vi "Test ReInit.vi"(7 "Sequence Context In":refnum<k7>, 8 "error in":errorcluster, 9 "Test Mode":u16, 10 "LV PPS Config":T1={"VISA Resource"="", "Voltage Level (0.0 V)"=12.0, "CURRent Limit (0.0 A)"=6.0, "OVP LEVEL (0V)"=15.0, "Enable OVP (T: Enable)"=FALSE, "OCP LEVEL (0A)"=8.0, "Enable OCP (T: Enable)"=TRUE, "Value Out"="", "Value In"="", "Actual Voltage Level (V)"=-0.11, "Actual Current Limit (A)"=0.0, "Select Instrument"="", "Enable Output"=TRUE, "PPS Operation"=enum."Configure", "Type"=0} {"Type" items=["Voltage", "Current"]; "Actual Current Limit (A)" format="%.2f"; "Actual Voltage Level (V)" format="%.2f"; "OCP LEVEL (0A)" format="%.2f"; "OVP LEVEL (0V)" format="%.2f"; "Voltage Level (0.0 V)" format="%.2f"}, 11 "HV PPS Config":T1={"VISA Resource"="", "Voltage Level (0.0 V)"=48.0, "CURRent Limit (0.0 A)"=150.0, "OVP LEVEL (0V)"=55.0, "Enable OVP (T: Enable)"=FALSE, "OCP LEVEL (0A)"=160.0, "Enable OCP (T: Enable)"=TRUE, "Value Out"="", "Value In"="", "Actual Voltage Level (V)"=-0.11, "Actual Current Limit (A)"=0.0, "Select Instrument"="", "Enable Output"=TRUE, "PPS Operation"=enum."Configure", "Type"=0} {"Type" items=["Voltage", "Current"]; "Actual Current Limit (A)" format="%.2f"; "Actual Voltage Level (V)" format="%.2f"; "OCP LEVEL (0A)" format="%.2f"; "OVP LEVEL (0V)" format="%.2f"; "Voltage Level (0.0 V)" format="%.2f"}) -> (0 "error out":errorcluster, 2 "Response Code":u8[](array[numeric]), 3 "Positive Responce":bool)   [LabVIEW 2023, in "HardwareAbstractionLayer_LVOOP.lvlib" / "Wait Monitor.lvclass"]
uses:
  Wait Monitor.lvclass
  PowerSupply/Teststand/Control/PPS StepType Control.ctl
  CAN/CAN Application Protocols/STP Protocol_class/Ctrls/STP CMD.ctl
  Teststand Steptypes/CAN/STP/Steptypes/Control/STP Data.ctl
  Teststand Steptypes/DAQ/Relay Output/Control/Relay Output.ctl
  069355f8-7d87-48c7-8f90-e89c4997140f.vi
  3c8db822-b366-47eb-99a2-87ce3c109eb2.vi
  f5ace3f9-55e8-4b56-8f2c-1356bb897dc4.vi
  57b82cc3-dd7c-4d3a-8ba9-81b38abffcad.vi
  725d82db-e125-4af1-8c31-2eddca650097.vi
  e56fdc52-0104-40be-a5d4-315e7d7fad48.vi
  ae1cdcb4-d38d-44ac-ba66-047396e49866.vi
  Teststand/Teststand.lvclass
  PowerSupply/PowerSupply.lvclass
  CAN/CAN Application Protocols/STP Protocol_class/STP Protocol.lvclass
  Teststand Steptypes/LTT_TeststandSteptypes.lvlib
  b7294423-ed5d-4e5b-8d0b-fca4433a2c56.vi
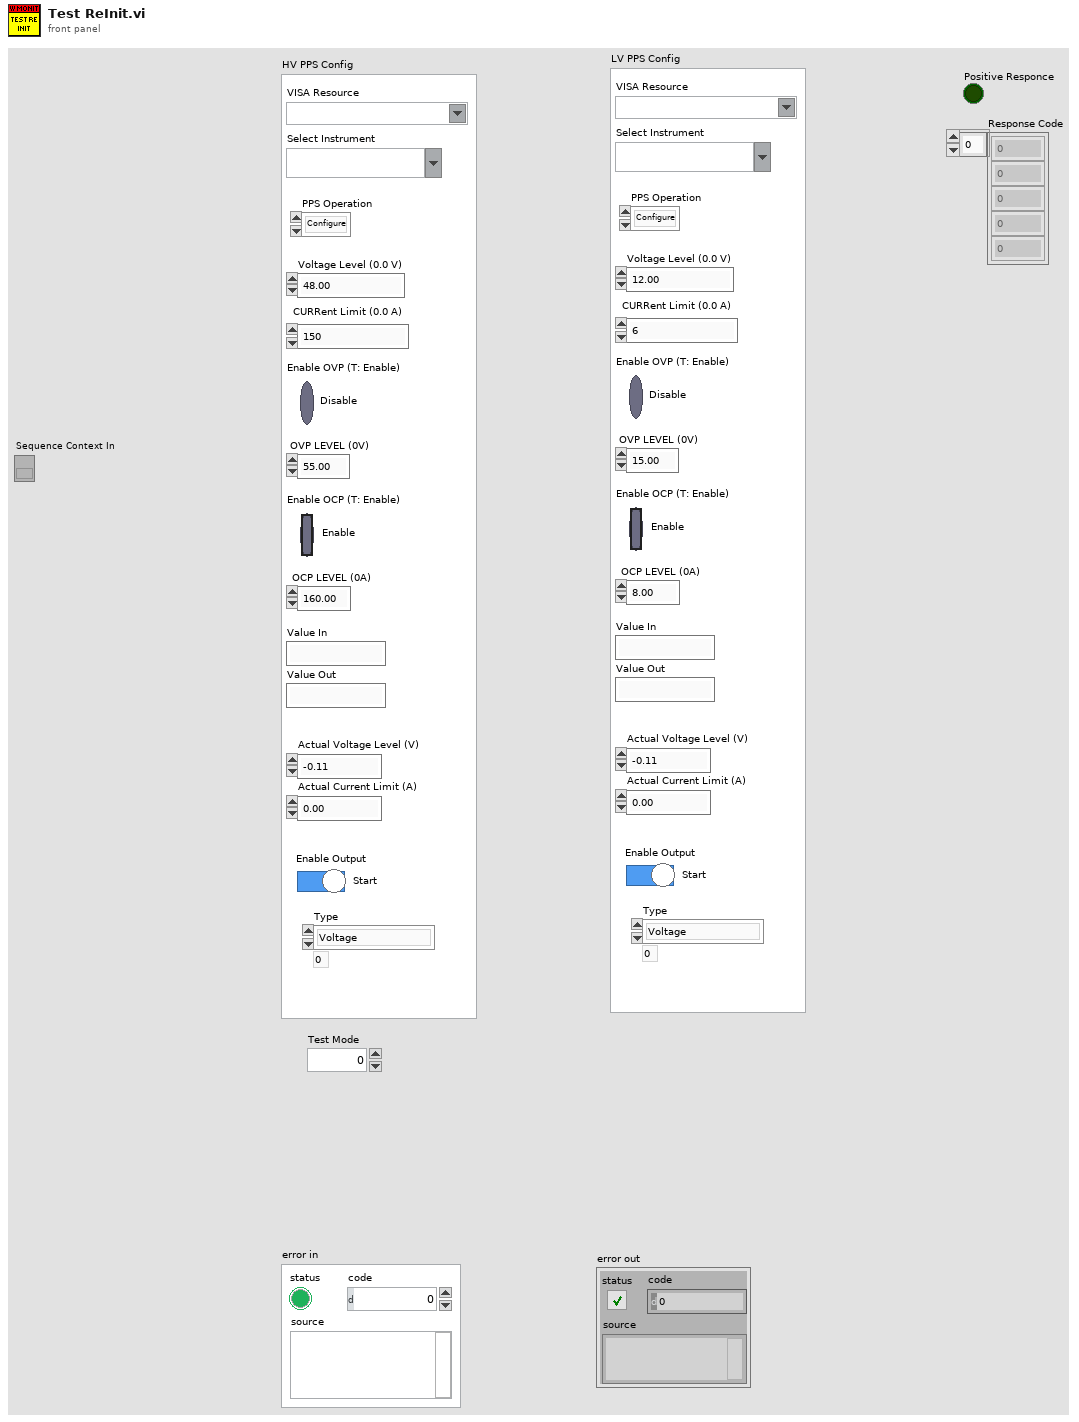
[diagram p1: front panel]
types:
  T1 = typedef "HardwareAbstractionLayer_LVOOP.lvlib/PowerSupply.lvclass/PPS StepType Control.ctl" = cluster{"VISA Resource":refnum<visa-resource-name>, "Voltage Level (0.0 V)":dbl, "CURRent Limit (0.0 A)":dbl, "OVP LEVEL (0V)":dbl, "Enable OVP (T: Enable)":bool, "OCP LEVEL (0A)":dbl, "Enable OCP (T: Enable)":bool, "Value Out":string, "Value In":string, "Actual Voltage Level (V)":dbl, "Actual Current Limit (A)":dbl, "Select Instrument":string, "Enable Output":bool, "PPS Operation":enum32{"Init", "Self Test", "Configure", "Measure", "Close"}, "Type":u16}
  T2 = enum32{"Init", "Self Test", "Configure", "Measure", "Close"}
  T3 = typedef "LTT_TeststandSteptypes.lvlib/STP Data.ctl" = cluster{"ECU CAN Port":string, "CMD":T4, "CAN Write Data":u8[], "Response Decoder":enum16{"String", "Number", "Boolean"}, "String":cluster{"Start Index":i32, "Length":i32}, "Number":cluster{"MSB Index":i32, "LSB Index":i32}, "Boolean":cluster{"Index":i32, "Bool":cluster{"7":bool, "6":bool, "5":bool, "4":bool, "3":bool, "2":bool, "1":bool, "0":bool, "7 Enabled":bool, "6 Enabled":bool, "5 Enabled":bool, "4 Enabled":bool, "3 Enabled":bool, "2 Enabled":bool, "1 Enabled":bool, "0 Enabled":bool}}}
  T4 = typedef "HardwareAbstractionLayer_LVOOP.lvlib/CAN Application Protocols Lib.lvlib/STP Protocol.lvclass/STP CMD.ctl" = u8
  T5 = typedef "LTT_TeststandSteptypes.lvlib/Relay Output.ctl" = cluster{"Signal Name List":cluster{"Signal Name":string, "Enable Output":bool}[]}
  T6 = typedef "HardwareAbstractionLayer_LVOOP.lvlib/Teststand.lvclass/Teststand Status Control.ctl" = cluster{"Terminating or Aborting":bool, "Stop":bool, "Socket Count":i16, "Selected Sockets":i16[]}
  T7 = typedef "LTT_TeststandSteptypes.lvlib/STP Out Data.ctl" = cluster{"String Data":string, "Numeric Data":dbl, "Boolean Data":bool, "RequestTimeout?":bool, "ResponseData":u8[], "PositiveResponse?":bool}
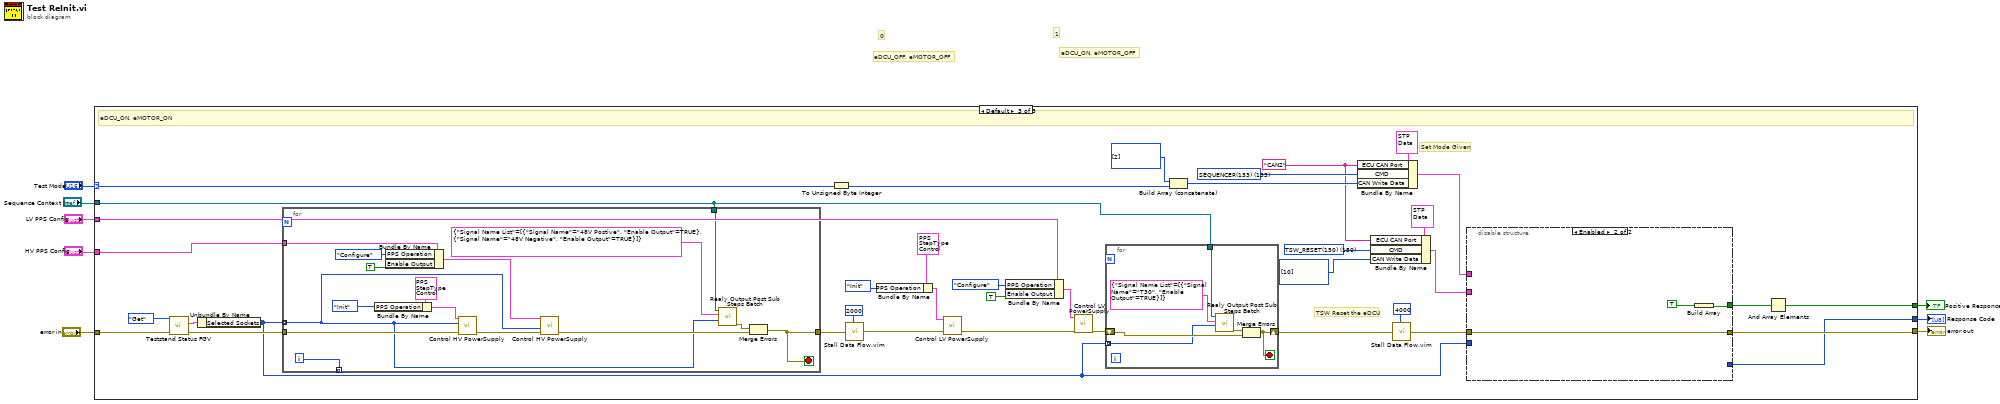
[diagram p0: block diagram]
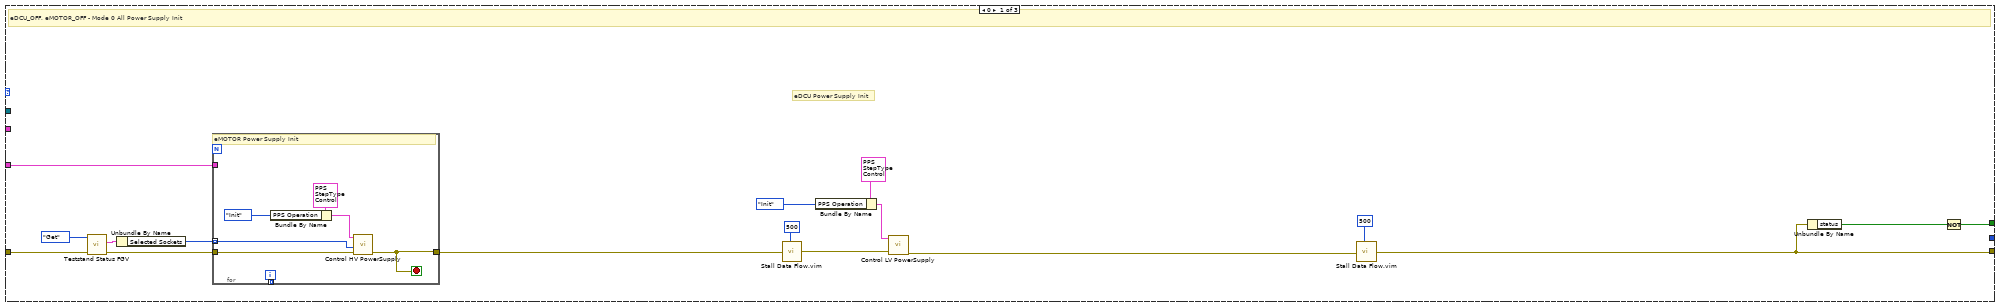
[diagram p2: hidden frame]
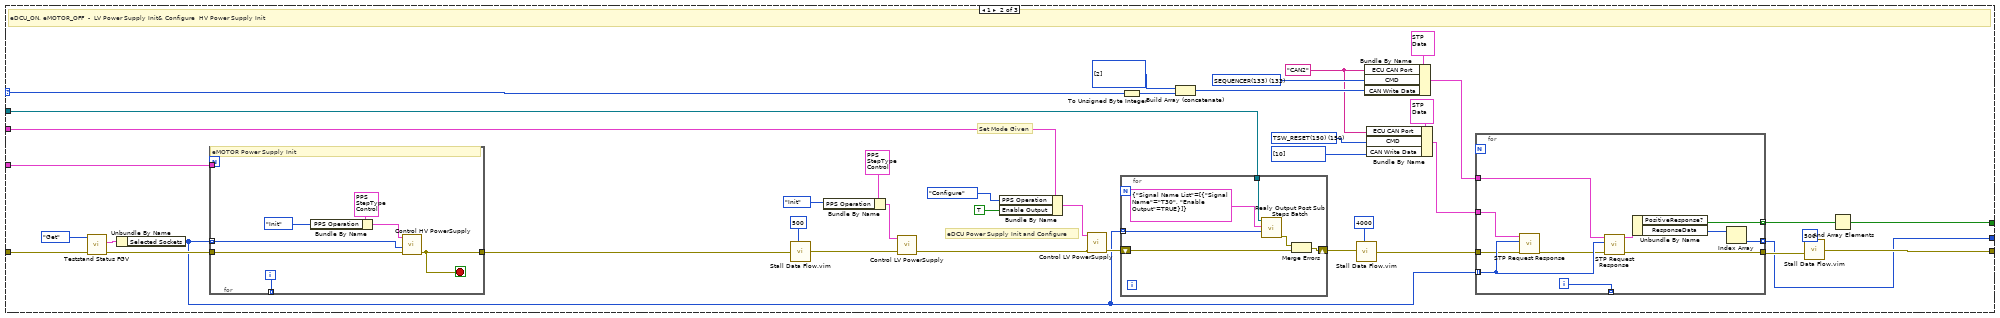
[diagram p3: hidden frame]
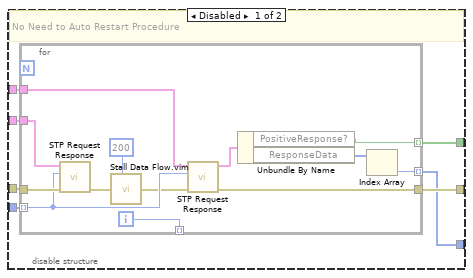
[diagram p4: hidden frame]
diagram:
  # "0"
  # "1"
  # "eDCU_ON, eMOTOR_OFF"
  # "eDCU_OFF, eMOTOR_OFF"
  n1 = case shown="Default" "Test Mode" {
    selector: "Test Mode" -> [_ w54 w116]
    tunnel: "error in" -> [w22 w69 w131]
    tunnel: [w11 w50 w122] -> w7
    tunnel: "HV PPS Config" -> [w21 w68 w130]
    tunnel: "LV PPS Config" -> [_ w63 w125]
    tunnel: [w10 w48 w112] -> w3
    tunnel: [_ w47 w111] -> w2
    tunnel: "Sequence Context In" -> [_ w38 w103]
    frame 0 {
      # "eDCU Power Supply Init"
      # "eDCU_OFF, eMOTOR_OFF - Mode 0 All Power Supply Init"
      n2 = call "Teststand Status FGV.vi"("error in"=w22, "Option"=enum16{"Set", "Get"}."Get") -> ("error out"=w23:errorcluster, "Teststand Status Out"=w24:T6)  [unwired: 8 in]
      n3 = Unbundle By Name(w24) -> ("Selected Sockets"=w15:i16[])
      n4 = for {
        tunnel: w23 -> [w31]
        tunnel: [w30] -> w20
        tunnel: w15 -> [w32] mode=indexing
        tunnel: w21 -> [_]
        tunnel: [w26] -> _ mode=indexing
        i -> [w26]
        stop <- w30 stop-if-true
        # "eMOTOR Power Supply Init"
        n5 = Bundle By Name(cluster=T1 {"VISA Resource"="", "Voltage Level (0.0 V)"=0.0, "CURRent Limit (0.0 A)"=0.0, "OVP LEVEL (0V)"=0.0, "Enable OVP (T: Enable)"=TRUE, "OCP LEVEL (0A)"=0.0, "Enable OCP (T: Enable)"=TRUE, "Value Out"="", "Value In"="", "Actual Voltage Level (V)"=0.0, "Actual Current Limit (A)"=0.0, "Select Instrument"="", "Enable Output"=FALSE, "PPS Operation"=enum."Init", "Type"=0} ("PPS Config In"), "PPS Operation"=T2."Init") -> (w27:T1)
        n6 = call "Control HV PowerSupply.vi"("error in"=w31, "Socket Index"=w32, "PPS Config In"=w27) -> ("error out"=w30:errorcluster)  [unwired: 6 in, 2 out]
      }
      n7 = call "Stall Data Flow.vim"("value in"=w20, "milliseconds to wait"=u32 500) -> ("value out"=w13:errorcluster)  [unwired: 1 out]
      n8 = Bundle By Name(cluster=T1 {"VISA Resource"="", "Voltage Level (0.0 V)"=12.0, "CURRent Limit (0.0 A)"=6.0, "OVP LEVEL (0V)"=15.0, "Enable OVP (T: Enable)"=FALSE, "OCP LEVEL (0A)"=8.0, "Enable OCP (T: Enable)"=TRUE, "Value Out"="", "Value In"="", "Actual Voltage Level (V)"=-0.11, "Actual Current Limit (A)"=0.0, "Select Instrument"="", "Enable Output"=TRUE, "PPS Operation"=enum."Init", "Type"=0} ("PPS Config In"), "PPS Operation"=T2."Init") -> (w14:T1)
      n9 = call "Control LV PowerSupply.vi"("error in"=w13, "PPS Config In"=w14) -> ("error out"=w12:errorcluster)  [unwired: 7 in, 2 out]
      n10 = call "Stall Data Flow.vim"("value in"=w12, "milliseconds to wait"=u32 500) -> ("value out"=w11:errorcluster)  [unwired: 1 out]
      n11 = Unbundle By Name(w11) -> ("status"=w9:bool)
      n12 = Not(x=w9) -> (.not. x?=w10:bool)
    }
    frame 1 {
      w36 = T4 150 items=["TSW_VERSION(130)"=130, "WAIT_EVENT(132)"=132, "SEQUENCER(133)"=133, "TSW_RESET(150)"=150, "CONFIG_ECU(151)"=151, "TEST_CORE (152)"=152, "TEST_WATCHDOG (153)"=153, "TEST_MONITORING (154)"=154, "READ_MEMORY (162)"=162, "WRITE_ERASE_MEMORY (164)"=164, "COMM_EXTERNAL (190)"=190, "COMM_INTERNAL (195)"=195, "GET_ANALOG_INPUT (210)"=210, "GET_DIGITAL_INPUT (211)"=211, "GET_FREQUENCY_INPUT (212)"=212, "TEST_INPUT_STRUCTURE (214)"=214, "GENERATE_OUTPUT_SIGNAL (220)"=220, "GENERATE_SYNCHRONIZED_OUTPUT_SIGNALS (221)"=221, "eDCU_Specific (250)"=250] ("CMD")
      w56 = T4 133 items=["TSW_VERSION(130)"=130, "WAIT_EVENT(132)"=132, "SEQUENCER(133)"=133, "TSW_RESET(150)"=150, "CONFIG_ECU(151)"=151, "TEST_CORE (152)"=152, "TEST_WATCHDOG (153)"=153, "TEST_MONITORING (154)"=154, "READ_MEMORY (162)"=162, "WRITE_ERASE_MEMORY (164)"=164, "COMM_EXTERNAL (190)"=190, "COMM_INTERNAL (195)"=195, "GET_ANALOG_INPUT (210)"=210, "GET_DIGITAL_INPUT (211)"=211, "GET_FREQUENCY_INPUT (212)"=212, "TEST_INPUT_STRUCTURE (214)"=214, "GENERATE_OUTPUT_SIGNAL (220)"=220, "GENERATE_SYNCHRONIZED_OUTPUT_SIGNALS (221)"=221, "eDCU_Specific (250)"=250] ("CMD")
      w35 = "CAN2" ("ECU CAN Port")
      # "eDCU Power Supply Init and Configure"
      # "Set Mode Given"
      # "eDCU_ON, eMOTOR_OFF  -  LV Power Supply Init& Configure  HV Power Supply Init"
      n13 = call "Teststand Status FGV.vi"("error in"=w69, "Option"=enum16{"Set", "Get"}."Get") -> ("error out"=w70:errorcluster, "Teststand Status Out"=w71:T6)  [unwired: 8 in]
      n14 = Unbundle By Name(w71) -> ("Selected Sockets"=w39:i16[])
      n15 = for {
        tunnel: w70 -> [w95]
        tunnel: [w94] -> w67
        tunnel: w39 -> [w96] mode=indexing
        tunnel: w68 -> [_]
        tunnel: [w90] -> _ mode=indexing
        i -> [w90]
        stop <- w94 stop-if-true
        # "eMOTOR Power Supply Init"
        n16 = Bundle By Name(cluster=T1 {"VISA Resource"="", "Voltage Level (0.0 V)"=0.0, "CURRent Limit (0.0 A)"=0.0, "OVP LEVEL (0V)"=0.0, "Enable OVP (T: Enable)"=TRUE, "OCP LEVEL (0A)"=0.0, "Enable OCP (T: Enable)"=TRUE, "Value Out"="", "Value In"="", "Actual Voltage Level (V)"=0.0, "Actual Current Limit (A)"=0.0, "Select Instrument"="", "Enable Output"=FALSE, "PPS Operation"=enum."Init", "Type"=0} ("PPS Config In"), "PPS Operation"=T2."Init") -> (w91:T1)
        n17 = call "Control HV PowerSupply.vi"("error in"=w95, "Socket Index"=w96, "PPS Config In"=w91) -> ("error out"=w94:errorcluster)  [unwired: 6 in, 2 out]
      }
      n18 = call "Stall Data Flow.vim"("value in"=w67, "milliseconds to wait"=u32 500) -> ("value out"=w45:errorcluster)  [unwired: 1 out]
      n19 = Bundle By Name(cluster=T1 {"VISA Resource"="", "Voltage Level (0.0 V)"=12.0, "CURRent Limit (0.0 A)"=6.0, "OVP LEVEL (0V)"=15.0, "Enable OVP (T: Enable)"=FALSE, "OCP LEVEL (0A)"=8.0, "Enable OCP (T: Enable)"=TRUE, "Value Out"="", "Value In"="", "Actual Voltage Level (V)"=-0.11, "Actual Current Limit (A)"=0.0, "Select Instrument"="", "Enable Output"=TRUE, "PPS Operation"=enum."Init", "Type"=0} ("PPS Config In"), "PPS Operation"=T2."Init") -> (w46:T1)
      n20 = call "Control LV PowerSupply.vi"("error in"=w45, "PPS Config In"=w46) -> ("error out"=w43:errorcluster)  [unwired: 7 in, 2 out]
      n21 = Bundle By Name(cluster=w63, "PPS Operation"=T2."Configure", "Enable Output"=TRUE) -> (w44:T1)
      n22 = call "Control LV PowerSupply.vi"("error in"=w43, "PPS Config In"=w44) -> ("error out"=w41:errorcluster)  [unwired: 7 in, 2 out]
      n23 = for {
        tunnel: w38 -> [w77]
        shift-right: [w75] -> w40
        shift-left: w41 -> [w76]
        tunnel: w39 -> [w73] mode=indexing
        n24 = call "Realy Output Post Sub Steps Batch.vi"("Socket No"=w73, "RelayOutputWrite"=T5 {"Signal Name List"=[{"Signal Name"="T30", "Enable Output"=TRUE}]}, "Sequence Context In"=w77) -> ("error out"=w74:errorcluster)  [unwired: 6 in, 2 out]
        n25 = Merge Errors(w74, w76) -> (w75:errorcluster)
      }
      n26 = To Unsigned Byte Integer(number=w54) -> (unsigned 8bit integer=w53:u8)
      n27 = Build Array (concatenate)(u8[] [2] ("CAN Write Data"), w53) -> (w52:u8[])
      n28 = call "Stall Data Flow.vim"("value in"=w40, "milliseconds to wait"=u32 4000) -> ("value out"=w59:errorcluster)  [unwired: 1 out]
      n29 = Bundle By Name(cluster=T3 {"ECU CAN Port"="CAN2", "CMD"=130, "CAN Write Data"=[], "Response Decoder"=enum."String", "String"={"Start Index"=0, "Length"=-1}, "Number"={"MSB Index"=0, "LSB Index"=1}, "Boolean"={"Index"=0, "Bool"={"7"=FALSE, "6"=FALSE, "5"=FALSE, "4"=FALSE, "3"=FALSE, "2"=FALSE, "1"=FALSE, "0"=FALSE, "7 Enabled"=FALSE, "6 Enabled"=FALSE, "5 Enabled"=FALSE, "4 Enabled"=FALSE, "3 Enabled"=FALSE, "2 Enabled"=FALSE, "1 Enabled"=FALSE, "0 Enabled"=FALSE}}} ("STP Data in"), "ECU CAN Port"=w35, "CMD"=w56, "CAN Write Data"=w52) -> (w57:T3)
      n30 = Bundle By Name(cluster=T3 {"ECU CAN Port"="CAN2", "CMD"=130, "CAN Write Data"=[], "Response Decoder"=enum."String", "String"={"Start Index"=0, "Length"=-1}, "Number"={"MSB Index"=0, "LSB Index"=1}, "Boolean"={"Index"=0, "Bool"={"7"=FALSE, "6"=FALSE, "5"=FALSE, "4"=FALSE, "3"=FALSE, "2"=FALSE, "1"=FALSE, "0"=FALSE, "7 Enabled"=FALSE, "6 Enabled"=FALSE, "5 Enabled"=FALSE, "4 Enabled"=FALSE, "3 Enabled"=FALSE, "2 Enabled"=FALSE, "1 Enabled"=FALSE, "0 Enabled"=FALSE}}} ("STP Data in"), "ECU CAN Port"=w35, "CMD"=w36, "CAN Write Data"=u8[] [10]) -> (w33:T3)
      n31 = for {
        tunnel: w57 -> [w88]
        tunnel: [w87] -> _ mode=indexing
        tunnel: w39 -> [w82] mode=indexing
        tunnel: w59 -> [w80]
        tunnel: [w89] -> w60
        tunnel: [w85] -> w51 mode=indexing
        tunnel: [w83] -> w47 mode=indexing
        tunnel: w33 -> [w81]
        i -> [w87]
        n32 = call "STP Request Response.vi"("error in"=w80, "Socket No"=w82, "STP Data in"=w81) -> ("error out"=w79:errorcluster)  [unwired: 5 in, 3 out]
        n33 = call "STP Request Response.vi"("error in"=w79, "Socket No"=w82, "STP Data in"=w88) -> ("error out"=w89:errorcluster, "STP Data Out"=w86:T7)  [unwired: 5 in, 2 out]
        n34 = Unbundle By Name(w86) -> ("PositiveResponse?"=w85:bool, "ResponseData"=w84:u8[])
        n35 = Index Array(array=w84) -> (element=w83:u8)  [unwired: 1 in]
      }
      n36 = call "Stall Data Flow.vim"("value in"=w60, "milliseconds to wait"=u32 500) -> ("value out"=w50:errorcluster)  [unwired: 1 out]
      n37 = And Array Elements(Boolean array=w51) -> (logical AND=w48:bool)
    }
    frame Default {
      w100 = T4 150 items=["TSW_VERSION(130)"=130, "WAIT_EVENT(132)"=132, "SEQUENCER(133)"=133, "TSW_RESET(150)"=150, "CONFIG_ECU(151)"=151, "TEST_CORE (152)"=152, "TEST_WATCHDOG (153)"=153, "TEST_MONITORING (154)"=154, "READ_MEMORY (162)"=162, "WRITE_ERASE_MEMORY (164)"=164, "COMM_EXTERNAL (190)"=190, "COMM_INTERNAL (195)"=195, "GET_ANALOG_INPUT (210)"=210, "GET_DIGITAL_INPUT (211)"=211, "GET_FREQUENCY_INPUT (212)"=212, "TEST_INPUT_STRUCTURE (214)"=214, "GENERATE_OUTPUT_SIGNAL (220)"=220, "GENERATE_SYNCHRONIZED_OUTPUT_SIGNALS (221)"=221, "eDCU_Specific (250)"=250] ("CMD")
      w118 = T4 133 items=["TSW_VERSION(130)"=130, "WAIT_EVENT(132)"=132, "SEQUENCER(133)"=133, "TSW_RESET(150)"=150, "CONFIG_ECU(151)"=151, "TEST_CORE (152)"=152, "TEST_WATCHDOG (153)"=153, "TEST_MONITORING (154)"=154, "READ_MEMORY (162)"=162, "WRITE_ERASE_MEMORY (164)"=164, "COMM_EXTERNAL (190)"=190, "COMM_INTERNAL (195)"=195, "GET_ANALOG_INPUT (210)"=210, "GET_DIGITAL_INPUT (211)"=211, "GET_FREQUENCY_INPUT (212)"=212, "TEST_INPUT_STRUCTURE (214)"=214, "GENERATE_OUTPUT_SIGNAL (220)"=220, "GENERATE_SYNCHRONIZED_OUTPUT_SIGNALS (221)"=221, "eDCU_Specific (250)"=250] ("CMD")
      w97 = "CAN2" ("ECU CAN Port")
      # "TSW Reset the eDCU"
      # "Set Mode Given"
      # "eDCU_ON, eMOTOR_ON"
      n38 = call "Teststand Status FGV.vi"("error in"=w131, "Option"=enum16{"Set", "Get"}."Get") -> ("error out"=w132:errorcluster, "Teststand Status Out"=w133:T6)  [unwired: 8 in]
      n39 = Unbundle By Name(w133) -> ("Selected Sockets"=w102:i16[])
      n40 = for {
        tunnel: w132 -> [w175]
        tunnel: [w166] -> w129
        tunnel: w102 -> [w164] mode=indexing
        tunnel: w130 -> [w178]
        tunnel: [w170] -> _ mode=indexing
        tunnel: w103 -> [w167]
        i -> [w170]
        stop <- w166 stop-if-true
        n41 = Bundle By Name(cluster=T1 {"VISA Resource"="", "Voltage Level (0.0 V)"=0.0, "CURRent Limit (0.0 A)"=0.0, "OVP LEVEL (0V)"=0.0, "Enable OVP (T: Enable)"=TRUE, "OCP LEVEL (0A)"=0.0, "Enable OCP (T: Enable)"=TRUE, "Value Out"="", "Value In"="", "Actual Voltage Level (V)"=0.0, "Actual Current Limit (A)"=0.0, "Select Instrument"="", "Enable Output"=FALSE, "PPS Operation"=enum."Init", "Type"=0} ("PPS Config In"), "PPS Operation"=T2."Init") -> (w171:T1)
        n42 = Bundle By Name(cluster=w178, "PPS Operation"=T2."Configure", "Enable Output"=TRUE) -> (w177:T1)
        n43 = call "Control HV PowerSupply.vi"("error in"=w175, "Socket Index"=w164, "PPS Config In"=w171) -> ("error out"=w174:errorcluster)  [unwired: 6 in, 2 out]
        n44 = call "Control HV PowerSupply.vi"("error in"=w174, "Socket Index"=w164, "PPS Config In"=w177) -> ("error out"=w179:errorcluster)  [unwired: 6 in, 2 out]
        n45 = call "Realy Output Post Sub Steps Batch.vi"("Socket No"=w164, "RelayOutputWrite"=T5 {"Signal Name List"=[{"Signal Name"="48V Postive", "Enable Output"=TRUE}, {"Signal Name"="48V Negative", "Enable Output"=TRUE}]}, "Sequence Context In"=w167) -> ("error out"=w165:errorcluster)  [unwired: 6 in, 2 out]
        n46 = Merge Errors(w165, w179) -> (w166:errorcluster)
      }
      n47 = To Unsigned Byte Integer(number=w116) -> (unsigned 8bit integer=w115:u8)
      n48 = call "Stall Data Flow.vim"("value in"=w129, "milliseconds to wait"=u32 2000) -> ("value out"=w109:errorcluster)  [unwired: 1 out]
      n49 = Bundle By Name(cluster=T1 {"VISA Resource"="", "Voltage Level (0.0 V)"=12.0, "CURRent Limit (0.0 A)"=6.0, "OVP LEVEL (0V)"=15.0, "Enable OVP (T: Enable)"=FALSE, "OCP LEVEL (0A)"=8.0, "Enable OCP (T: Enable)"=TRUE, "Value Out"="", "Value In"="", "Actual Voltage Level (V)"=-0.11, "Actual Current Limit (A)"=0.0, "Select Instrument"="", "Enable Output"=TRUE, "PPS Operation"=enum."Init", "Type"=0} ("PPS Config In"), "PPS Operation"=T2."Init") -> (w110:T1)
      n50 = call "Control LV PowerSupply.vi"("error in"=w109, "PPS Config In"=w110) -> ("error out"=w107:errorcluster)  [unwired: 7 in, 2 out]
      n51 = Bundle By Name(cluster=w125, "PPS Operation"=T2."Configure", "Enable Output"=TRUE) -> (w108:T1)
      n52 = call "Control LV PowerSupply.vi"("error in"=w107, "PPS Config In"=w108) -> ("error out"=w104:errorcluster)  [unwired: 7 in, 2 out]
      n53 = for {
        shift-right: [w158] -> w105
        shift-left: w104 -> [w161]
        tunnel: w103 -> [w160]
        tunnel: w102 -> [w159] mode=indexing
        stop <- w158 stop-if-true
        n54 = call "Realy Output Post Sub Steps Batch.vi"("Socket No"=w159, "RelayOutputWrite"=T5 {"Signal Name List"=[{"Signal Name"="T30", "Enable Output"=TRUE}]}, "Sequence Context In"=w160) -> ("error out"=w162:errorcluster)  [unwired: 6 in, 2 out]
        n55 = Merge Errors(w162, w161) -> (w158:errorcluster)
      }
      n56 = Build Array (concatenate)(u8[] [2] ("CAN Write Data"), w115) -> (w114:u8[])
      n57 = Bundle By Name(cluster=T3 {"ECU CAN Port"="CAN2", "CMD"=130, "CAN Write Data"=[], "Response Decoder"=enum."String", "String"={"Start Index"=0, "Length"=-1}, "Number"={"MSB Index"=0, "LSB Index"=1}, "Boolean"={"Index"=0, "Bool"={"7"=FALSE, "6"=FALSE, "5"=FALSE, "4"=FALSE, "3"=FALSE, "2"=FALSE, "1"=FALSE, "0"=FALSE, "7 Enabled"=FALSE, "6 Enabled"=FALSE, "5 Enabled"=FALSE, "4 Enabled"=FALSE, "3 Enabled"=FALSE, "2 Enabled"=FALSE, "1 Enabled"=FALSE, "0 Enabled"=FALSE}}} ("STP Data in"), "ECU CAN Port"=w97, "CMD"=w118, "CAN Write Data"=w114) -> (w119:T3)
      n58 = Bundle By Name(cluster=T3 {"ECU CAN Port"="CAN2", "CMD"=130, "CAN Write Data"=[], "Response Decoder"=enum."String", "String"={"Start Index"=0, "Length"=-1}, "Number"={"MSB Index"=0, "LSB Index"=1}, "Boolean"={"Index"=0, "Bool"={"7"=FALSE, "6"=FALSE, "5"=FALSE, "4"=FALSE, "3"=FALSE, "2"=FALSE, "1"=FALSE, "0"=FALSE, "7 Enabled"=FALSE, "6 Enabled"=FALSE, "5 Enabled"=FALSE, "4 Enabled"=FALSE, "3 Enabled"=FALSE, "2 Enabled"=FALSE, "1 Enabled"=FALSE, "0 Enabled"=FALSE}}} ("STP Data in"), "ECU CAN Port"=w97, "CMD"=w100, "CAN Write Data"=u8[] [10]) -> (w98:T3)
      n59 = call "Stall Data Flow.vim"("value in"=w105, "milliseconds to wait"=u32 4000) -> ("value out"=w121:errorcluster)  [unwired: 1 out]
      n60 = disable-structure shown="Enabled" {
        disable-tunnel: [w141 w157] -> w122
        disable-tunnel: w121 -> [w140 w157]
        disable-tunnel: w119 -> [w139 _]
        disable-tunnel: [w138 w155] -> w113
        disable-tunnel: [w137 _] -> w111
        disable-tunnel: w102 -> [w136 _]
        disable-tunnel: w98 -> [w135 _]
        frame Disabled {
          # "No Need to Auto Restart Procedure"
          n61 = for {
            tunnel: w139 -> [w153]
            tunnel: [w152] -> _ mode=indexing
            tunnel: w136 -> [w144] mode=indexing
            tunnel: w140 -> [w147]
            tunnel: [w154] -> w141
            tunnel: [w150] -> w138 mode=indexing
            tunnel: [w148] -> w137 mode=indexing
            tunnel: w135 -> [w145]
            i -> [w152]
            n62 = call "STP Request Response.vi"("error in"=w147, "Socket No"=w144, "STP Data in"=w145) -> ("error out"=w146:errorcluster)  [unwired: 5 in, 3 out]
            n63 = call "Stall Data Flow.vim"("value in"=w146, "milliseconds to wait"=u32 200) -> ("value out"=w143:errorcluster)  [unwired: 1 out]
            n64 = call "STP Request Response.vi"("error in"=w143, "Socket No"=w144, "STP Data in"=w153) -> ("error out"=w154:errorcluster, "STP Data Out"=w151:T7)  [unwired: 5 in, 2 out]
            n65 = Unbundle By Name(w151) -> ("PositiveResponse?"=w150:bool, "ResponseData"=w149:u8[])
            n66 = Index Array(array=w149) -> (element=w148:u8)  [unwired: 1 in]
          }
        }
        frame Enabled {
          n67 = Build Array(TRUE) -> (w155:bool[])
        }
      }
      n68 = And Array Elements(Boolean array=w113) -> (logical AND=w112:bool)
    }
  }
  "error out" <- w7
  "Positive Responce" <- w3
  "Response Code" <- w2
